vi "Resettable Trigger.vi"(8 "error in (no error)":errorcluster, 9 "Reset (F)":bool, 10 "State":bool) -> (0 "error out":errorcluster, 1 "Triggered?":bool, 2 "Trigger":bool)   [LabVIEW 2012]
doc: "This VI sets the \"Trigger\" output high only once on a rising edge of the \"State\" input. The \"Triggered?\" output is high after the first time there is a rising edge on the \"State\" input. The trigger is resettable through the input \"Reset (F)\".\n\nFreeware from Moore Good Ideas, www.mooregoodideas.com. Do not remove this line."
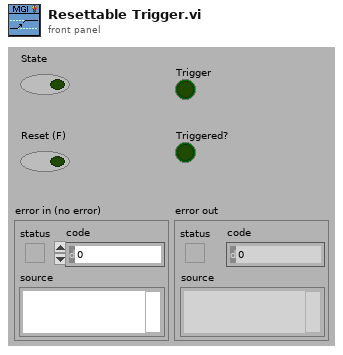
[diagram p1: front panel]
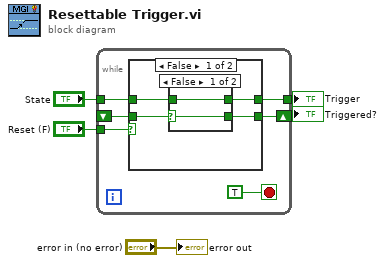
[diagram p0: block diagram]
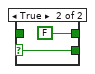
[diagram p2: hidden frame]
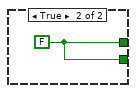
[diagram p3: hidden frame]
diagram:
  n1 = while {
    tunnel: "State" -> [w8]
    shift-right: [w10] -> w1
    shift-left: _ -> [w9]
    tunnel: [w7] -> w4
    tunnel: "Reset (F)" -> [w6]
    stop <- TRUE stop-if-true
    n2 = case shown="False" w6 {
      tunnel: [w14 w19] -> w10
      tunnel: w9 -> [w13 _]
      tunnel: w8 -> [w15 _]
      tunnel: [w12 w19] -> w7
      frame False {
        n3 = case shown="False" w13 {
          selector: w13 -> [_ w18]
          tunnel: w15 -> [w16 _]
          tunnel: [w16 w18] -> w14
          tunnel: [w16 FALSE ("State")] -> w12
          frame False {
          }
          frame True {
          }
        }
      }
      frame True {
        w19 = FALSE ("State")
      }
    }
  }
  "Trigger" <- w4
  "Triggered?" <- w1
  "error out" <- "error in (no error)"
